vi "15.扫描引擎同步.vi"() -> ()   [LabVIEW 2019]
uses:
  <vilib>/rvi/Emulation/niFpgaGetClockAttributes.vi
  <vilib>/rvi/Emulation/niFpgaSctlEmulationGetInTimedLoop.vi
  <vilib>/rvi/Emulation/niFpgaEmulationReportErrorSimple.vi
  <vilib>/rvi/eio/common/nirviEmuTemplatePropertyGet_noerrors.vi
  <vilib>/rvi/Emulation/niFpgaCriticalErrorInLSC.vi
  <vilib>/rvi/eio/common/nirviEmuTemplateMethod_errors.vi
  <vilib>/eio/EIOPropertyNode/EIOPropertyNode.xnode
  <vilib>/eio/EIOMethodNode/EIOMethodNode.xnode
  <vilib>/rvi/eio/common/nirviEmuTemplatePropertyGet_errors.vi
  <vilib>/rvi/eio/common/nirviEmuTemplatePropertySet_errors.vi
  <vilib>/rvi/eio/common/nirviEmuTemplatePropertySet_noerrors.vi
panel:
  in  "停止":bool
  out "Missed Falling Edge":bool
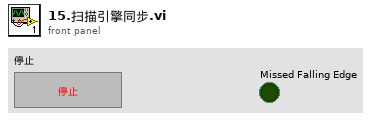
[diagram p1: front panel]
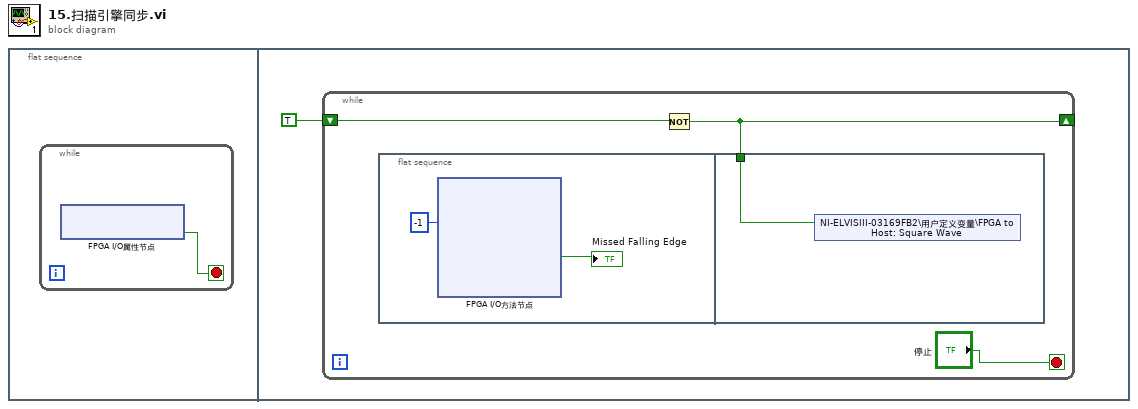
[diagram p0: block diagram]
diagram:
  n1 = flat-sequence {
    frame #0 {
      n2 = while {
        stop <- w1 stop-if-true
        n3 = xnode "FPGA I/O属性节点"() -> ("启用"=w1:bool)  [unwired: 1 in, 1 out]
      }
    }
    frame #1 {
      n4 = while {
        shift-right: [w4] -> _
        shift-left: TRUE -> [w5]
        stop <- "停止" stop-if-true
        n5 = flat-sequence {
          tunnel: w4 -> [w8]
          frame #0 {
            n6 = xnode "FPGA I/O方法节点"("超时"=-1) -> ("丢失的下降沿"=→"Missed Falling Edge":bool)  [unwired: 1 in, 4 out]
          }
          frame #1 {
            n7 = shared-variable "NI-ELVISIII-03169FB2\\用户定义变量\\FPGA to Host: Square Wave"(w8) -> ()  [unwired: 1 in, 1 out]
          }
        }
        n8 = Not(x=w5) -> (.not. x?=w4:bool)
      }
    }
  }
